vi "STL- STLToArray.vi"(8 "Boolean":bool, 10 "String":string, 11 "file (use dialog)":path) -> (2 "Array 3":dbl[][](array[numeric]))   [LabVIEW 2019]
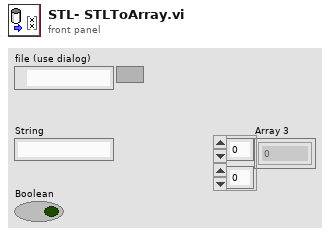
[diagram p1: front panel]
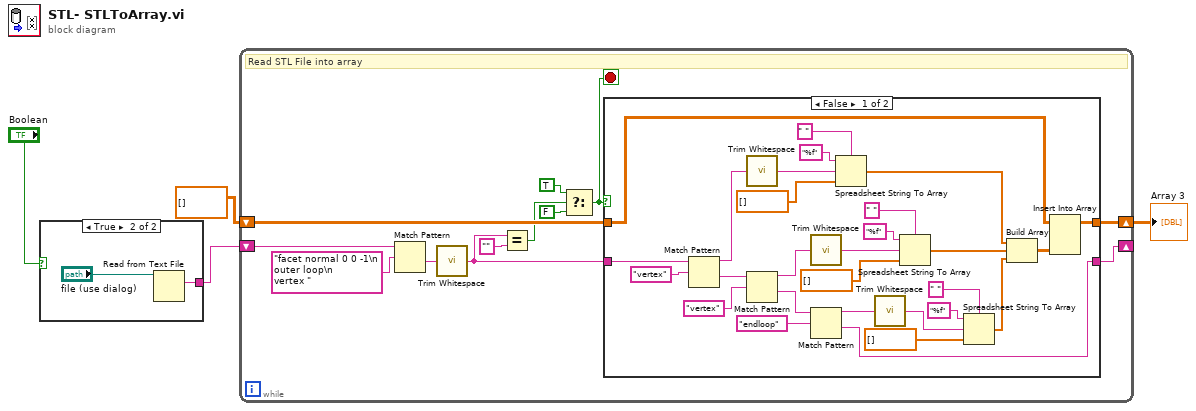
[diagram p0: block diagram]
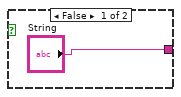
[diagram p2: hidden frame]
diagram:
  n1 = case shown="True" "Boolean" {
    tunnel: ["String" w6] -> w1
    frame False {
    }
    frame True {
      n2 = Read from Text File(file (use dialog)="file (use dialog)") -> (text=w6:string)  [unwired: 3 in, 3 out]
    }
  }
  n3 = while {
    shift-right: [w9] -> _
    shift-left: w1 -> [w17]
    shift-right: [w15] -> w4
    shift-left: dbl[][] [] ("Array 3") -> [w16]
    stop <- w8 stop-if-true
    # "Read STL File into array"
    n4 = Match Pattern(string=w17, regular expression="facet normal 0 0 -1\n    outer loop\n      vertex ") -> (after substring=w18:string)  [unwired: 1 in, 3 out]
    n5 = call <vilib>:"Trim Whitespace.vi"("string"=w18) -> ("trimmed string"=w14:string)  [unwired: 1 in]
    n6 = Equal?(x=w14, y="") -> (x = y?=w12:bool)
    n7 = Select(t=TRUE, s=w12, f=FALSE) -> (s? t:f=w8:bool)
    n8 = case shown="False" w8 {
      tunnel: w16 -> [w46 w48]
      tunnel: [w45 w48] -> w15
      tunnel: w14 -> [w44 w49]
      tunnel: [w21 w49] -> w9
      frame False {
        n9 = Match Pattern(string=w44, regular expression="vertex") -> (before substring=w39:string, after substring=w31:string)  [unwired: 1 in, 2 out]
        n10 = call <vilib>:"Trim Whitespace.vi"("string"=w39) -> ("trimmed string"=w38:string)  [unwired: 1 in]
        n11 = Match Pattern(string=w31, regular expression="vertex") -> (before substring=w33:string, after substring=w22:string)  [unwired: 1 in, 2 out]
        n12 = call <vilib>:"Trim Whitespace.vi"("string"=w33) -> ("trimmed string"=w32:string)  [unwired: 1 in]
        n13 = Match Pattern(string=w22, regular expression="endloop") -> (before substring=w24:string, after substring=w21:string)  [unwired: 1 in, 2 out]
        n14 = Spreadsheet String To Array(delimiter (Tab)=" ", format string="%f", spreadsheet string=w38, array type (2D Dbl)=dbl[] []) -> (array=w30:dbl[])
        n15 = call <vilib>:"Trim Whitespace.vi"("string"=w24) -> ("trimmed string"=w23:string)  [unwired: 1 in]
        n16 = Spreadsheet String To Array(delimiter (Tab)=" ", format string="%f", spreadsheet string=w32, array type (2D Dbl)=dbl[] []) -> (array=w29:dbl[])
        n17 = Spreadsheet String To Array(delimiter (Tab)=" ", format string="%f", spreadsheet string=w23, array type (2D Dbl)=dbl[] []) -> (array=w20:dbl[])
        n18 = Build Array(w30, w29, w20) -> (w47:dbl[][])
        n19 = Insert Into Array(array=w46, new element=w47) -> (w45:dbl[][])  [unwired: 2 in]
      }
      frame True {
      }
    }
  }
  "Array 3" <- w4
